vi "Clear - Core.vi"(8 "error in (no error)":errorcluster, 10 "Error Code":i32, 11 "Error Filter in":refnum<class "Error Filter.lvclass">) -> (0 "error out":errorcluster, 3 "Error Filter out":refnum<class "Error Filter.lvclass">)   [LabVIEW 2026, in "TALOS.lvlib" / "Classes.lvlib" / "Error Filter.lvclass"]
uses:
  Error Filter.lvclass
  Error Filter.lvclass/Error Filter.ctl
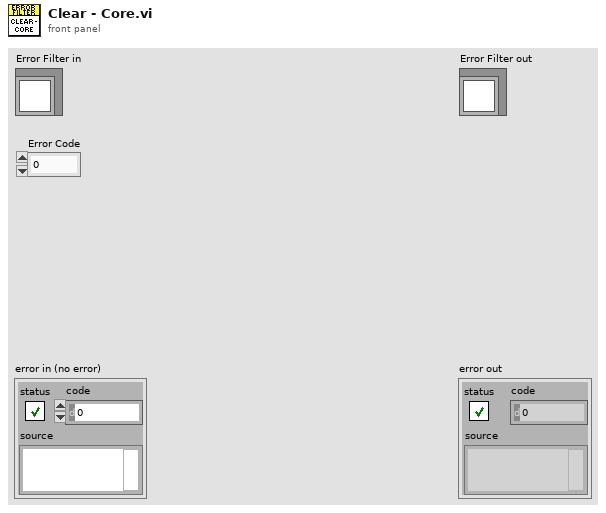
[diagram p1: front panel]
types:
  T1 = typedef "TALOS.lvlib/Classes.lvlib/Error Filter.lvclass/Error Filter Properties.ctl" = cluster{"Repetitions":u32, "Until":timestamp}
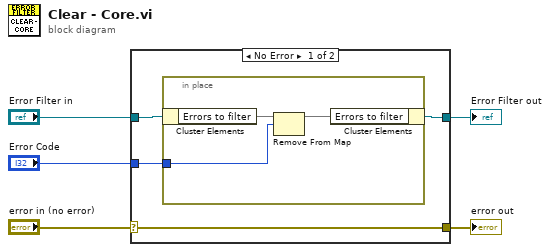
[diagram p0: block diagram]
diagram:
  n1 = case shown="No Error" "error in (no error)" {
    selector: "error in (no error)" -> [w9 w14]
    tunnel: [w9 w14] -> w4
    tunnel: [w6 w13] -> w2
    tunnel: "Error Filter in" -> [w8 w13]
    tunnel: "Error Code" -> [w7 _]
    frame No Error {
      n2 = in-place {
        in-place-border: w7 -> [w11]
        n3 = in-place-cluster #1(w8) -> ("Errors to filter"=w12:map{i32, T1})
        n4 = Remove From Map(10:w11, 11:w12) -> (3:w10:map{i32, T1})  [unwired: 2 out]
        n5 = in-place-cluster #1("Errors to filter"=w10) -> (w6:refnum<class "Error Filter.lvclass">)
      }
    }
    frame Error {
    }
  }
  "error out" <- w4
  "Error Filter out" <- w2
